vi "Intake Global.vi"() -> ()   [LabVIEW 2013]
panel:
  in  "Intake Info":T1
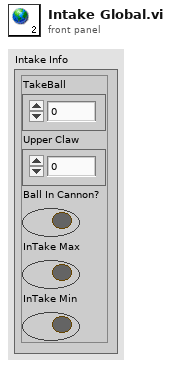
[diagram p1: front panel]
types:
  T1 = cluster{"TakeBall":dbl, "Upper Claw":dbl, "Ball In Cannon?":bool, "InTake Max":bool, "InTake Min":bool}
diagram:
